vi "Error list.vi"() -> (3 "regular expression":string[](array[string]))   [LabVIEW 2019]
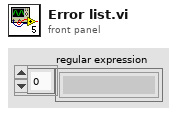
[diagram p1: front panel]
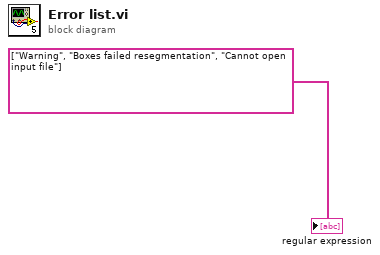
[diagram p0: block diagram]
diagram:
  "regular expression" <- string[] ["Warning", "Boxes failed resegmentation", "Cannot open input file"] ("regular expression")
